vi "Get Status String.vi"(8 "error in (no error)":errorcluster, 11 "Task in":refnum<class "Task.lvclass">) -> (0 "error out":errorcluster, 2 "Status":string, 3 "Task out":refnum<class "Task.lvclass">)   [LabVIEW 2017, in "Task Interface.lvlib" / "Task.lvclass"]
uses:
  Task.lvclass
  Task.lvclass/Task.ctl
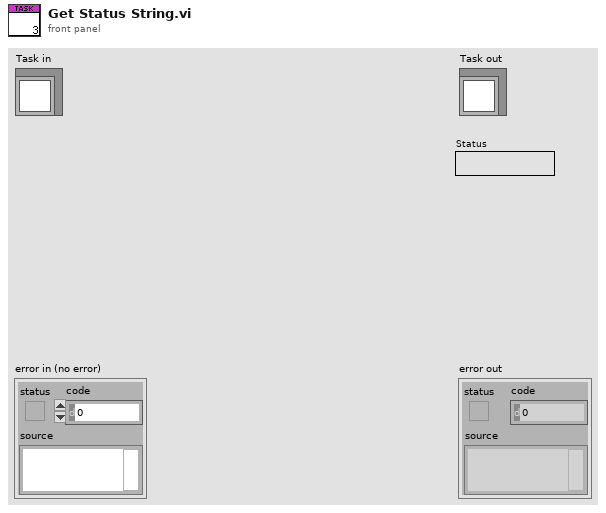
[diagram p1: front panel]
types:
  T1 = typedef "Task Interface.lvlib/Task.lvclass/Status.ctl" = enum16{"Created", "Added", "Pending", "Queued", "Processing", "Cleaning", "Building", "Finished", "Failed", "Removed", "Not found"}
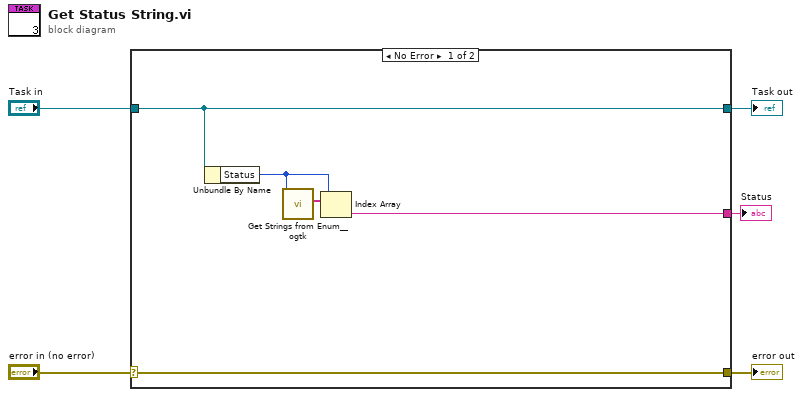
[diagram p0: block diagram]
diagram:
  n1 = case shown="No Error" "error in (no error)" {
    selector: "error in (no error)" -> [w10 w12]
    tunnel: [w10 w12] -> w4
    tunnel: [w8 w11] -> w2
    tunnel: "Task in" -> [w8 w11]
    tunnel: [w6 _] -> w1
    frame No Error {
      n2 = Unbundle By Name(w8) -> ("Status"=w7:T1)
      n3 = call <userlib>:"Get Strings from Enum__ogtk.vi"("Enum"=w7) -> ("Enum Strings"=w9:string[])  [unwired: 7 in, 3 out]
      n4 = Index Array(array=w9, index=w7) -> (element=w6:string)
    }
    frame Error {
    }
  }
  "error out" <- w4
  "Task out" <- w2
  "Status" <- w1
